vi "Read Message event.vi"(8 "error in (no error)":errorcluster, 11 "Mag Lab Measure Interface in":refnum<class "Mag Lab Measure UI.lvclass">) -> (0 "error out":errorcluster, 2 "Message event":refnum<user-event>, 3 "Mag Lab Measure Interface out":refnum<class "Mag Lab Measure UI.lvclass">)   [LabVIEW 2015, in "Mag Lab Measure UI.lvclass"]
uses:
  Mag Lab Measure UI.lvclass
  Mag Lab Measure UI.lvclass/Mag Lab Measure UI.ctl
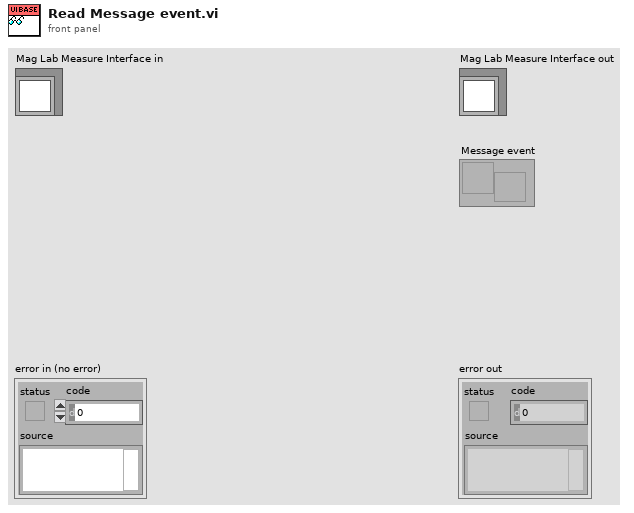
[diagram p1: front panel]
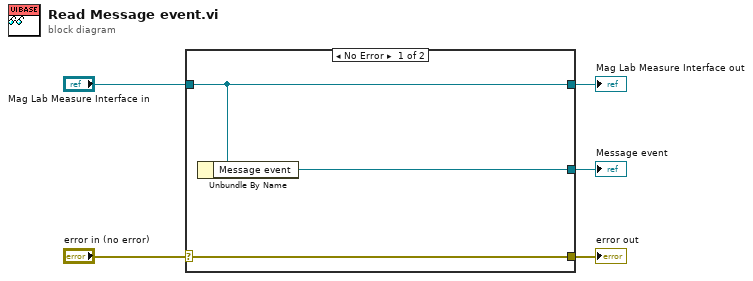
[diagram p0: block diagram]
diagram:
  n1 = case shown="No Error" "error in (no error)" {
    selector: "error in (no error)" -> [w8 w9]
    tunnel: [w8 w9] -> w4
    tunnel: [w7 w10] -> w2
    tunnel: "Mag Lab Measure Interface in" -> [w7 w10]
    tunnel: [w6 _] -> w1
    frame No Error {
      n2 = Unbundle By Name(w7) -> ("Message event"=w6:refnum<user-event>)
    }
    frame Error {
    }
  }
  "error out" <- w4
  "Mag Lab Measure Interface out" <- w2
  "Message event" <- w1
